vi "processdata.vi"(10 "oldrawin":i32, 11 "rawin":i32) -> (3 "rawout2":i32)   [LabVIEW 2017]
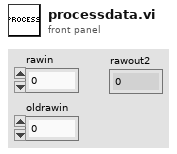
[diagram p1: front panel]
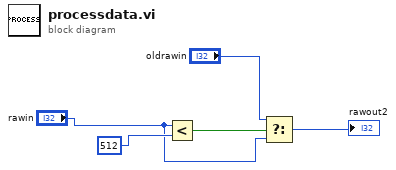
[diagram p0: block diagram]
diagram:
  n1 = Less?(x="rawin", y=512) -> (x < y?=w4:bool)
  n2 = Select(t="oldrawin", s=w4, f="rawin") -> (s? t:f=→"rawout2":i32)
